vi "List_TDMS Files_Generate AVI.vi"() -> ()   [LabVIEW 2017]
uses:
  Typedefs/Imaging Protocols enum.ctl
  Typedefs/ROI ID Enum.ctl
panel:
  in  "error in (no error)":errorcluster
  out "error out":errorcluster
  out "Number of  Trials":i32
  in  "Predominant ROI type":T1=enum."Comp. volume"
  in  "Imaging Protocol":T2=enum."Live Imaging"
  out "All Files in Dir":path[](array[path])
  in  "TDMS Folder Path":path
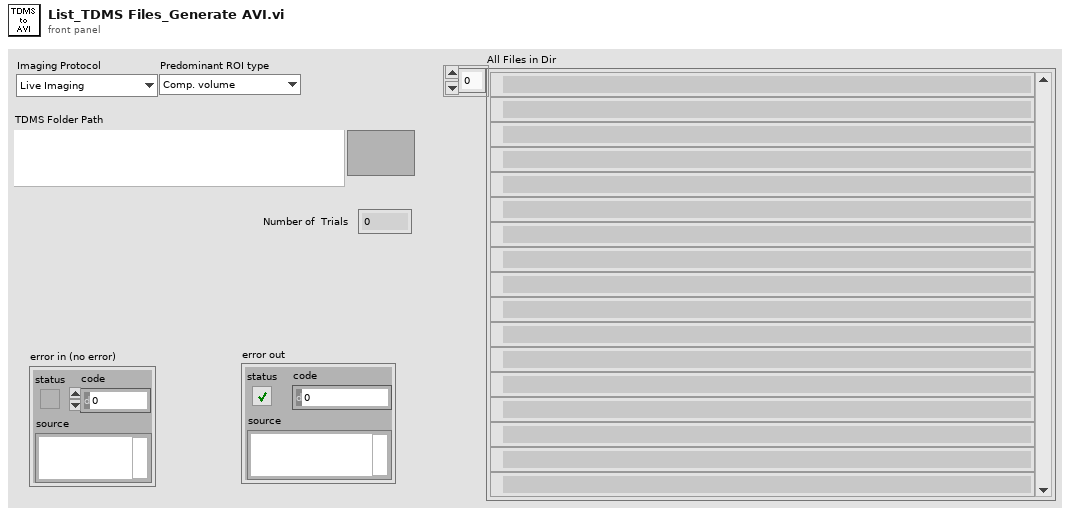
[diagram p1: front panel]
types:
  T1 = typedef "ROI ID Enum.ctl" = enum16{"Point", "MiniScan", "Comp. MiniScan", "Rectangle", "Comp. volume", "Arb. plane point"}
  T2 = typedef "Imaging Protocols enum.ctl" = enum16{"AOL Z-Stack", "Motor Z Stack", "Functional Acquisition", "Single Plane Acquisition", "Volume Acquisition", "Live Imaging", "Live Plane Imaging", "Live Volume Imaging"}
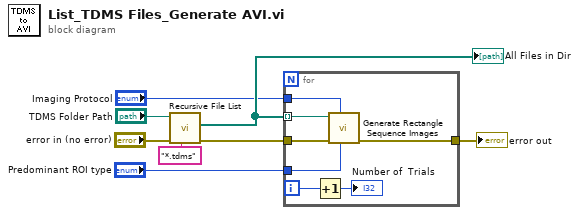
[diagram p0: block diagram]
diagram:
  n1 = call <vilib>:"Recursive File List.vi"("pattern"="*.tdms", "error in (no error)"="error in (no error)", "Folder Path"="TDMS Folder Path") -> ("error out"=w3:errorcluster, "All Files in Dir"=w6:path[])  [unwired: 4 in, 3 out]
  "All Files in Dir" <- w6
  n2 = for {
    tunnel: w6 -> [w14] mode=indexing
    tunnel: [w15] -> w2
    tunnel: "Imaging Protocol" -> [w13]
    tunnel: "Predominant ROI type" -> [w12]
    tunnel: w3 -> [w11]
    i -> [w10]
    n3 = Increment(x=w10) -> (x+1=→"Number of  Trials":i32)
    n4 = call "Generate Rectangle Sequence Images.vi"("Predominant ROI type"=w12, "Imaging Protocol"=w13, "error in (no error)"=w11, "TDMS file path & name"=w14) -> ("error out"=w15:errorcluster)  [unwired: 5 in, 2 out]
  }
  "error out" <- w2
